vi "PCO_SetMetaDataMode.vi"(8 "error in (no error)":errorcluster {"code" format="%x"}, 10 "wMetaDataMode":u16(ring) items=["OFF", "ON"], 11 "ph":u64) -> (0 "error out":errorcluster {"code" format="%x"}, 1 "wMetaDataSize":u16, 2 "ErrorMessage":i32 format="%x", 3 "ph out":u64, 5 "wMetaDataVersion":u16)   [LabVIEW 2019, in "SDK.lvlib" / "RecordingControl.lvlib"]
doc: "<b>Description:</b>\nThis function does to set the mode for Meta Data and returns information about size and version of the Meta Data block.\nWhen Meta Data mode is set to [on], a Meta Data block with additional information is added at the end of each image. The internal buffers allocated with PCO_AllocateBuffer are adapted automatically. If the buffers are allocated externally, the user is responsible to add further line(s), where the number of lines depends on horizontal resolution and the size of the additional Meta Data block.\nNote: Meta Data mode must not be changed during one session. Failure to follow this rule might result in an application crash.\n\n<b>Supported camera type:</b>\npco.dimax, pco.edge\n\n<b>Descriptor dependency:</b>\ndwGeneralCapsDESC1: METADATA"
uses:
  RecordingControl.lvlib
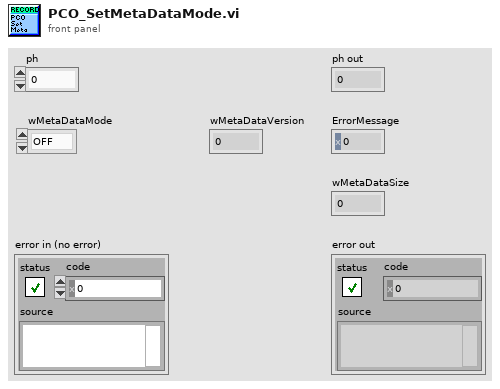
[diagram p1: front panel]
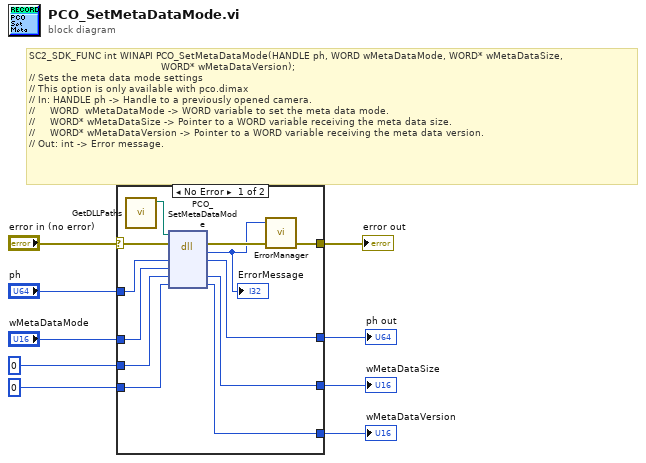
[diagram p0: block diagram]
diagram:
  # "SC2_SDK_FUNC int WINAPI PCO_SetMetaDataMode(HANDLE ph, WORD wMetaDataMode, WORD* wMetaDataSize,\n                                            WORD* wMetaDataVersion);\n// Sets the meta data mode settings\n// This option is only available with pco.dimax\n// In: HANDLE ph -> Handle to a previously opened camera.\n//     WORD  wMetaDataMode -> WORD variable to set the meta data mode.\n//     WORD* wMetaDataSize -> Pointer to a WORD variable receiving the meta data size.\n//     WORD* wMetaDataVersion -> Pointer to a WORD variable receiving the meta data version.\n// Out: int -> Error message."
  n1 = case shown="No Error" "error in (no error)" {
    selector: "error in (no error)" -> [w14 w25]
    tunnel: "ph" -> [w21 w24]
    tunnel: [w20 w24] -> w8
    tunnel: "wMetaDataMode" -> [w19 _]
    tunnel: u16 0 ("wMetaDataSize") -> [w18 w23]
    tunnel: [w17 w23] -> w5
    tunnel: u16 0 ("wMetaDataVersion") -> [w16 w22]
    tunnel: [w15 w22] -> w3
    tunnel: [w12 w25] -> w2
    frame No Error {
      n2 = call "GetDLLPaths.vi"() -> ("SC2_Cam_Path"=w10:path)  [unwired: 8 in, 3 out]
      n3 = dll-call lib="?" fn="PCO_SetMetaDataMode"(path in=w10, error in=w14, "ph"=w21, "wMetaDataMode"=w19, "wMetaDataSize"=w18, "wMetaDataVersion"=w16) -> (error out=w13:errorcluster, "return type"=w11:i32, "ph"=w20:u64, "wMetaDataSize"=w17:u16, "wMetaDataVersion"=w15:u16)  [unwired: 2 in, 1 out]
      "ErrorMessage" <- w11
      n4 = call "ErrorManager.vi"("error in (no error)"=w13, "error code"=w11) -> ("error out"=w12:errorcluster)  [unwired: 2 in, 1 out]
    }
    frame Error {
    }
  }
  "ph out" <- w8
  "wMetaDataSize" <- w5
  "wMetaDataVersion" <- w3
  "error out" <- w2
